vi "Sample Averaging.vi"(10 "Sample In":dbl[](array[numeric]), 11 "Averaging":bool) -> (3 "Sample Out":dbl[](array[numeric]))   [LabVIEW 2009]
panel:
  out "Number of Samples":u32
  out "Sums":dbl[](array[numeric])
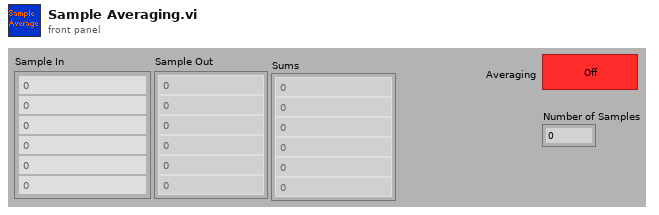
[diagram p1: front panel]
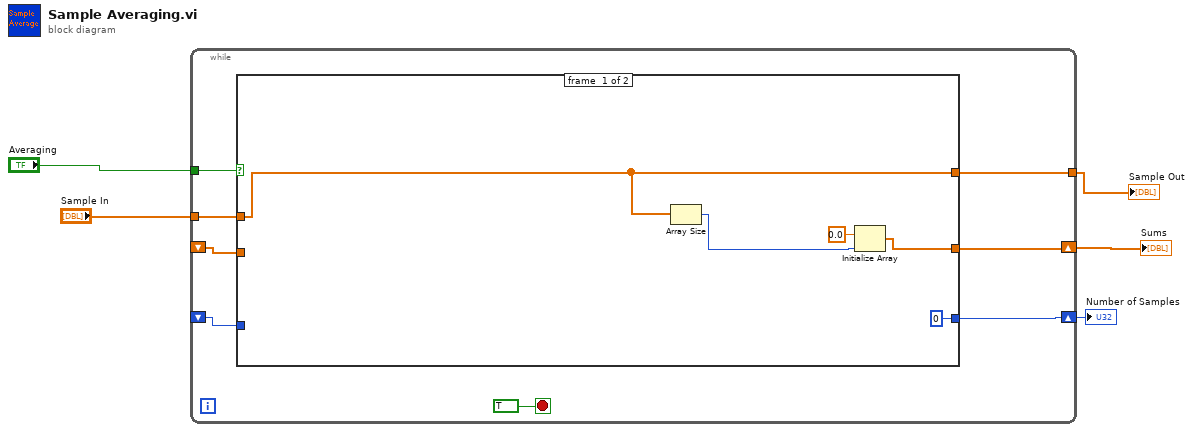
[diagram p0: block diagram]
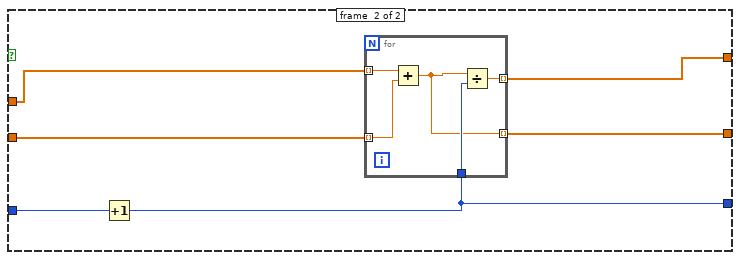
[diagram p2: hidden frame]
diagram:
  n1 = while {
    tunnel: "Averaging" -> [w12]
    shift-right: [w10] -> w2
    shift-left: _ -> [w11]
    tunnel: [w9] -> w5
    tunnel: "Sample In" -> [w8]
    shift-right: [w6] -> w1
    shift-left: _ -> [w7]
    stop <- TRUE stop-if-true
    n2 = case shown="False" w12 {
      tunnel: w11 -> [_ w23]
      tunnel: [w17 w19] -> w10
      tunnel: [w15 w24] -> w9
      tunnel: w8 -> [w15 w22]
      tunnel: w7 -> [_ w21]
      tunnel: [u32 0 w20] -> w6
      frame #0 {
        n3 = Array Size(array=w15) -> (size(s)=w14:i32)
        n4 = Initialize Array(0.0 ("element"), w14) -> (w17:dbl[])
      }
      frame #1 {
        n5 = Increment(x=w21) -> (x+1=w20:u32)
        n6 = for {
          tunnel: [w29] -> w24 mode=indexing
          tunnel: w23 -> [w28] mode=indexing
          tunnel: w22 -> [w27] mode=indexing
          tunnel: w20 -> [w26]
          tunnel: [w25] -> w19 mode=indexing
          n7 = Add(x=w27, y=w28) -> (x+y=w25:dbl)
          n8 = Divide(x=w25, y=w26) -> (x/y=w29:dbl)
        }
      }
    }
  }
  "Sample Out" <- w5
  "Sums" <- w2
  "Number of Samples" <- w1
